vi "peis.vi"(0 "IP adress":string="192.109.209.229", 1 "stop":bool, 2 "Channel":u8(ring) items=["1", "2", "3", "4", "5", "6", "7", "8", "9", "10", "11", "12", "13", "14", "15", "16"], 3 "PEIS Parameters":T2={"Step_number"=0, "Initial_Voltage_step"=0.0, "vs_initial"=TRUE, "Final_Voltage_step"=1.0, "vs_final"=FALSE, "Duration_step"=1.0, "Record_every_dI"=0.1, "Record_every_dT"=0.1, "Initial_frequency"=100000.0, "sweep"=FALSE, "Final_frequency"=1.0, "Frequency_number"=51, "Amplitude_Voltage"=0.01, "Wait_for_steady"=2.0, "Average_N_times"=1, "Correction"=TRUE, "I_Range"=12, "Bandwidth"=5, "em"=1, "ce"=0} {"ce" items=["Standard", "CE to ground"]; "Initial_Voltage_step" min=-10 max=10 format="%.5f"; "Step_number" min=0 step=1; "I_Range" items=["1pA", "1nA", "10nA", "100nA", "1µA", "10µA", "100µA", "1mA", "10mA", "100mA", "1A", "Booster", "Auto"]; "Wait_for_steady" min=0 format="%.2f"; "Record_every_dT" min=0 format="%.2e"; "Record_every_dI" min=0 format="%.2e"; "Duration_step" min=0 format="%.5f"; "Final_Voltage_step" min=-10 max=10 format="%.5f"; "Bandwidth" items=["1"=1, "2"=2, "3"=3, "4"=4, "5"=5, "6"=6, "7"=7, "8"=8, "9"=9]; "Average_N_times" min=1 max=1000 step=1; "Amplitude_Voltage" min=0.0005 max=0.5 format="%.2e"; "Final_frequency" min=1e-05 max=1000000 format="%.2e"; "Frequency_number" min=1 max=10000; "Initial_frequency" min=1e-05 max=1000000 format="%.2e"}, 4 "Exit":bool, 5 "Start":bool, 8 "Draw":T1(ring)) -> (6 "XY Graph":cluster{"Data p1":sgl[], "Data p1":dbl[]}[](graph), 7 "Number of points":i32=52)   [LabVIEW 2016]
doc: "The Staircase Potentio Electrochemical Impedance Spectroscopy (SPEIS) technique is designed to perform successive impedance measurements (on a whole frequency range) during a potential sweep. \nThis technique consists in a staircase potential sweep (potential limits and number of steps defined by the user). An impedance measurement (with an adjustable number of frequencies) is performed on each potential step.\n\nIn general, in this VI, the first thing to do is to start by establishing the connection with the instrument defined by its IP adress, then load the firmware in the channel selected, get the information on the plugged channels, load protocol on a channel, start/stop the protocol, retreive data and draw the graph.\nThis technique is applied just for channels with impedance capabilities (Zboard)."
uses:
  LLB/dll_Functions.llb/PEISParameters.ctl
panel:
  in  "Display Parameters?":bool caption="Display Parameters"
  out "DllPath":path caption="DLL Path"
  out "LibVersion":string caption="DLL Version"
  out "Data p0":sgl[][](array[numeric])=[[0.100008, 0.099745475, 1.9343544e-05], [0.200016, 0.09966919, 1.936642e-05], [0.300024, 0.10005063, 1.9374045e-05], [0.400032, 0.10005063, 1.9358795e-05], [0.50004, 0.09997434, 1.9358795e-05], [0.600048, 0.09982177, 1.938167e-05], [0.700056, 0.099516615, 1.9358795e-05], [0.800064, 0.099898055, 1.9374045e-05], [0.90007204, 0.099516615, 1.936642e-05]]
  out "Data p1":sgl[][](array[numeric])=[[99999.99, 0.009897927, 1.5485124e-05, -0.23932889, 0.09957624, 2.0601647e-05, 0.0, 0.017584162, 1.5528842e-05, -0.13801742, -0.10928005, -2.0601661e-05, 0.0, 1.89, 7.0], [79789.055, 0.009909321, 1.4999416e-05, -0.28277892, 0.09956935, 2.0610883e-05, 0.0, 0.017358849, 1.5026583e-05, -0.16497254, -0.10927754, -2.0610896e-05, 0.0, 2.319, 7.0], [63671.867, 0.00993305, 1.4371862e-05, -0.3338619, 0.099571265, 2.0617736e-05, 0.0, 0.01701651, 1.4388475e-05, -0.19887781, -0.10927467, -2.0617748e-05, 0.0, 2.748, 7.0], [50804.684, 0.009895762, 1.349999e-05, -0.38682938, 0.099595726, 2.0621628e-05, 0.0, 0.016509676, 1.3509973e-05, -0.23511207, -0.10929042, -2.0621641e-05, 0.0, 3.177, 7.0], [40539.06, 0.009924297, 1.2531375e-05, -0.43154812, 0.09956674, 2.0623062e-05, 0.0, 0.01605967, 1.2537333e-05, -0.27001935, -0.1092824, -2.0623074e-05, 0.0, 3.606, 7.0], [32343.752, 0.009929493, 1.1422184e-05, -0.4605673, 0.099575475, 2.0627644e-05, 0.0, 0.015497766, 1.1425662e-05, -0.29694676, -0.10927959, -2.0627656e-05, 0.0, 4.035, 7.0], [25812.496, 0.009931898, 1.0332502e-05, -0.47349262, 0.09957423, 2.0616248e-05, 0.0, 0.014982226, 1.0334525e-05, -0.31350675, -0.10928383, -2.0616259e-05, 0.0, 4.4639997, 7.0], [20593.748, 0.009683827, 9.104932e-06, -0.46709442, 0.09957324, 2.0613099e-05, 0.0, 0.014134236, 9.106069e-06, -0.3174526, -0.10928545, -2.0613114e-05, 0.0, 4.75, 7.0], [16429.69, 0.00984061, 8.381006e-06, -0.4425385, 0.0995779, 2.0614962e-05, 0.0, 0.013980997, 8.381673e-06, -0.30736777, -0.10928426, -2.0614974e-05, 0.0, 5.036, 7.0], [13109.373, 0.009880392, 7.759602e-06, -0.4042132, 0.09956233, 2.0629059e-05, 0.0, 0.013766184, 7.759997e-06, -0.28469434, -0.10927877, -2.0629072e-05, 0.0, 5.322, 7.0], [10460.936, 0.009915135, 7.290463e-06, -0.35881066, 0.099576354, 2.062228e-05, 0.0, 0.013552605, 7.2907023e-06, -0.25464892, -0.10927802, -2.0622294e-05, 0.0, 5.608, 7.0], [8351.5625, 0.009958473, 6.968417e-06, -0.30687237, 0.09957134, 2.0619169e-05, 0.0, 0.013452288, 6.968562e-06, -0.21966934, -0.10928822, -2.0619183e-05, 0.0, 5.894, 7.0], [6660.1553, 0.009773157, 6.585265e-06, -0.26302314, 0.09957721, 2.0628519e-05, 0.0, 0.013077308, 6.5853465e-06, -0.18975565, -0.109301746, -2.0628531e-05, 0.0, 6.0620003, 7.0], [5313.953, 0.009875495, 6.4977903e-06, -0.21722555, 0.09959636, 2.061105e-05, 0.0, 0.013129692, 6.497844e-06, -0.15612268, -0.10930546, -2.0611064e-05, 0.0, 6.269, 7.0], [4241.786, 0.009916322, 6.4091464e-06, -0.17841792, 0.09959986, 2.0643229e-05, 0.0, 0.013149473, 6.4091746e-06, -0.12683374, -0.109303646, -2.0643243e-05, 0.0, 6.4830003, 7.0], [3385.4163, 0.009962957, 6.371731e-06, -0.15283132, 0.09959816, 2.0641255e-05, 0.0, 0.013166811, 6.371748e-06, -0.11219756, -0.10930573, -2.0641268e-05, 0.0, 6.697, 7.0], [2699.3184, 0.009985389, 6.3324687e-06, -0.12883663, 0.099599674, 2.0642745e-05, 0.0, 0.013169419, 6.3324833e-06, -0.09362733, -0.10931173, -2.0642758e-05, 0.0, 6.9110003, 7.0], [2153.4448, 0.009996085, 6.3133293e-06, -0.11305499, 0.09959159, 2.0643656e-05, 0.0, 0.013185124, 6.313335e-06, -0.08275235, -0.109307505, -2.064367e-05, 0.0, 7.125, 7.0], [1717.748, 0.010014333, 6.2567524e-06, -0.10080016, 0.09959457, 2.0655203e-05, 0.0, 0.013182044, 6.256763e-06, -0.07431483, -0.10931141, -2.0655216e-05, 0.0, 7.34, 7.0], [1372.1951, 0.010016238, 6.2877625e-06, -0.09321749, 0.09959682, 2.064688e-05, 0.0, 0.013175669, 6.2877634e-06, -0.06877315, -0.10931128, -2.0646892e-05, 0.0, 7.5550003, 7.0], [1096.7545, 0.010012516, 6.286433e-06, -0.08541584, 0.09960139, 2.0640491e-05, 0.0, 0.013178928, 6.2864306e-06, -0.062073976, -0.10930484, -2.0640506e-05, 0.0, 7.77, 7.0], [871.93097, 0.010010969, 6.268487e-06, -0.08781743, 0.09959833, 2.0634905e-05, 0.0, 0.013172707, 6.2684835e-06, -0.06440747, -0.109307244, -2.0634918e-05, 0.0, 7.987, 7.0], [696.1138, 0.01003125, 6.2508416e-06, -0.093888, 0.09959319, 2.0650714e-05, 0.0, 0.013164024, 6.2508466e-06, -0.069969416, -0.10931639, -2.0650728e-05, 0.0, 8.203, 7.0], [555.8894, 0.010025321, 6.2520185e-06, -0.10746312, 0.099596396, 2.063822e-05, 0.0, 0.01315077, 6.2520166e-06, -0.08037281, -0.109306626, -2.0638234e-05, 0.0, 8.42, 7.0], [443.43906, 0.010033136, 6.209101e-06, -0.12175393, 0.0995993, 2.0631758e-05, 0.0, 0.01312816, 6.2091035e-06, -0.091670275, -0.109299496, -2.063177e-05, 0.0, 8.639, 7.0], [353.75473, 0.01003465, 6.1840165e-06, -0.14335668, 0.09959073, 2.0645593e-05, 0.0, 0.013097799, 6.1840187e-06, -0.10758209, -0.10931424, -2.0645608e-05, 0.0, 8.859, 7.0], [281.8943, 0.010030967, 6.109471e-06, -0.17281115, 0.09959446, 2.0650212e-05, 0.0, 0.013065848, 6.109473e-06, -0.129511, -0.10930905, -2.0650225e-05, 0.0, 9.0789995, 7.0], [225.3606, 0.010023677, 6.0119432e-06, -0.20512176, 0.09959748, 2.064375e-05, 0.0, 0.013001974, 6.0119396e-06, -0.15545309, -0.1093129, -2.0643763e-05, 0.0, 9.301, 7.0], [180.28844, 0.010028235, 5.913567e-06, -0.25207758, 0.0995884, 2.0643136e-05, 0.0, 0.012923154, 5.913563e-06, -0.19031943, -0.1093126, -2.0643149e-05, 0.0, 9.526, 7.0], [143.75787, 0.010025335, 5.723294e-06, -0.2980666, 0.09959362, 2.0638052e-05, 0.0, 0.012791262, 5.7232987e-06, -0.22673774, -0.109312676, -2.0638066e-05, 0.0, 9.755, 7.0], [114.59661, 0.0100282775, 5.478785e-06, -0.36026663, 0.09959826, 2.0642558e-05, 0.0, 0.012615283, 5.4787893e-06, -0.27884817, -0.109307505, -2.0642572e-05, 0.0, 9.987, 7.0], [91.552734, 0.010020258, 5.1631105e-06, -0.41180015, 0.09958356, 2.0632298e-05, 0.0, 0.012400166, 5.1631077e-06, -0.32256132, -0.10930771, -2.0632311e-05, 0.0, 10.219, 7.0], [72.87778, 0.010045694, 4.7920767e-06, -0.47027957, 0.0995903, 1.9318108e-05, 0.0, 0.012195916, 4.7920753e-06, -0.37585485, -0.10930665, -1.931812e-05, 0.0, 10.735, 6.0], [58.30223, 0.010017018, 4.3459513e-06, -0.5196618, 0.09958969, 1.931711e-05, 0.0, 0.011869716, 4.345951e-06, -0.41790736, -0.109305374, -1.9317124e-05, 0.0, 10.989, 6.0], [46.50297, 0.010043655, 3.8964367e-06, -0.5461425, 0.09958527, 1.9321726e-05, 0.0, 0.011661541, 3.8964395e-06, -0.45622373, -0.10929812, -1.9321737e-05, 0.0, 11.24, 6.0], [36.95101, 0.0100237075, 3.4589034e-06, -0.55786407, 0.09959118, 1.9322812e-05, 0.0, 0.011445447, 3.4589052e-06, -0.47548974, -0.1093029, -1.9322824e-05, 0.0, 11.498, 6.0], [29.592804, 0.010024518, 3.0782626e-06, -0.5442606, 0.099590674, 1.9320825e-05, 0.0, 0.011281099, 3.0782635e-06, -0.4723431, -0.10930497, -1.9320838e-05, 0.0, 11.782001, 6.0], [23.588463, 0.010025413, 2.7635026e-06, -0.50970626, 0.09959939, 1.931987e-05, 0.0, 0.011168829, 2.7635024e-06, -0.45203626, -0.10930516, -1.9319881e-05, 0.0, 12.092, 6.0], [18.780045, 0.010028319, 2.5114025e-06, -0.46162716, 0.0995976, 1.9318664e-05, 0.0, 0.01109292, 2.5114036e-06, -0.4128492, -0.109315775, -1.9318675e-05, 0.0, 12.425, 6.0], [15.024037, 0.010029642, 2.331001e-06, -0.4064955, 0.099582985, 1.9321948e-05, 0.0, 0.01104459, 2.3310024e-06, -0.36793888, -0.10930361, -1.9321958e-05, 0.0, 12.772, 6.0], [11.982363, 0.010013976, 2.1986236e-06, -0.3445742, 0.0995901, 1.9318428e-05, 0.0, 0.01101896, 2.198625e-06, -0.31417423, -0.10929007, -1.931844e-05, 0.0, 13.119, 6.0], [9.574144, 0.010021789, 2.1110484e-06, -0.29042864, 0.09959056, 1.931938e-05, 0.0, 0.011009957, 2.1110482e-06, -0.26570365, -0.10930588, -1.9319392e-05, 0.0, 13.55, 6.0], [7.6293964, 0.010015764, 2.047544e-06, -0.2358973, 0.09959619, 1.9324216e-05, 0.0, 0.010986972, 2.0475438e-06, -0.21676749, -0.10930043, -1.9324229e-05, 0.0, 14.088, 6.0], [6.084501, 0.010008753, 2.0095065e-06, -0.19609833, 0.09960107, 1.9321422e-05, 0.0, 0.010978085, 2.0095063e-06, -0.17923641, -0.10930903, -1.9321435e-05, 0.0, 14.758, 6.0], [4.858519, 0.0100127505, 1.9834858e-06, -0.15383446, 0.099605374, 1.9325236e-05, 0.0, 0.01099137, 1.983485e-06, -0.14275539, -0.10930968, -1.9325249e-05, 0.0, 15.594, 6.0], [3.8752477, 0.010018873, 1.964741e-06, -0.12660927, 0.09960577, 1.9319072e-05, 0.0, 0.01098087, 1.9647398e-06, -0.11773729, -0.10930894, -1.9319084e-05, 0.0, 16.639, 6.0], [3.1001983, 0.01002199, 1.954336e-06, -0.101673305, 0.09960291, 1.9318823e-05, 0.0, 0.010977447, 1.9543347e-06, -0.09406805, -0.10931086, -1.9318833e-05, 0.0, 17.943, 6.0], [2.4660668, 0.010017678, 1.9471984e-06, -0.08063111, 0.09960053, 1.9318097e-05, 0.0, 0.010982101, 1.9471975e-06, -0.07494378, -0.10931104, -1.9318108e-05, 0.0, 19.579, 6.0], [1.9649143, 0.01001538, 1.9460967e-06, -0.064157724, 0.09960199, 1.9316354e-05, 0.0, 0.010980325, 1.946096e-06, -0.06017399, -0.1093061, -1.9316365e-05, 0.0, 21.627, 6.0], [1.5725644, 0.010012327, 1.941652e-06, -0.051375534, 0.09960348, 1.9317453e-05, 0.0, 0.010977772, 1.9416514e-06, -0.04843211, -0.10930792, -1.9317464e-05, 0.0, 24.183, 6.0], [1.2520034, 0.010019626, 1.939335e-06, -0.041469768, 0.09961237, 1.9318904e-05, 0.0, 0.010981496, 1.9393347e-06, -0.038478374, -0.109313786, -1.9318915e-05, 0.0, 27.391, 6.0], [1.0016024, 0.010014649, 1.938777e-06, -0.033258826, 0.09960662, 1.931856e-05, 0.0, 0.010977961, 1.9387764e-06, -0.031450033, -0.109310396, -1.9318572e-05, 0.0, 31.398, 6.0]]
  out "Exit 2":bool=TRUE
  # "Instructions:\nBefore running the VI you must type a valid IP adress that corresponds to the instrument.Then press the Run button to execute this VI.\nWhile this VI is running, choose the available channel, enter the SPEIS parameters or keep the default\n values, then press the start button to begin the experience. \nChoose the waveform to draw : Nyquist, modZ, theta...\nPress the stop button to end experience and the exit button to stop the VI execution."
  # "Set E (V)  vs. previous"
  # "Before EIS  stay for ts (s)"
  # "and record every dI (A)"
  # "or every dt (s)"
  # "Start EIS from  Fi (Hz)"
  # "sweep linear/logarithmic"
  # "to Ff (Hz)"
  # "for Nf frequencies"
  # "with the amplitude (V)"
  # "wait for Pw"
  # "average Na times"
  # "drift correction"
  # "with I Range"
  # "and bandwidth"
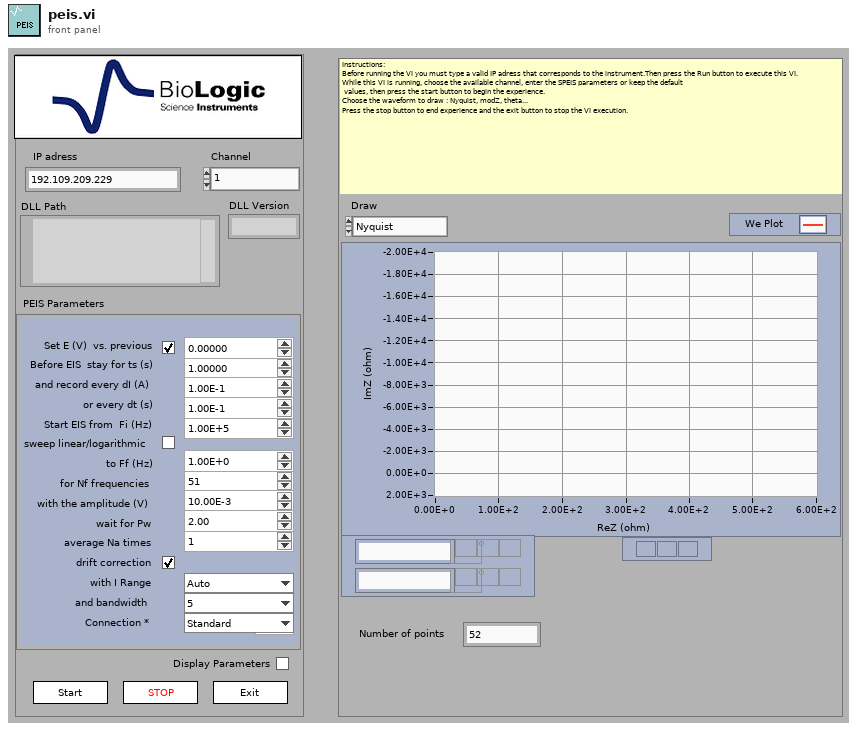
[diagram p1: front panel]
types:
  T1 = enum16{"Nyquist", "modZ", "theta", "modE", "modI", "Edc", "Idc", "E range", "I range", "f(t)"}
  T2 = typedef "PEISParameters.ctl" = cluster{"Step_number":i32, "Initial_Voltage_step":sgl, "vs_initial":bool, "Final_Voltage_step":sgl, "vs_final":bool, "Duration_step":sgl, "Record_every_dI":sgl, "Record_every_dT":sgl, "Initial_frequency":sgl, "sweep":bool, "Final_frequency":sgl, "Frequency_number":i32, "Amplitude_Voltage":sgl, "Wait_for_steady":sgl, "Average_N_times":i32, "Correction":bool, "I_Range":u16, "Bandwidth":u16, "em":u16, "ce":u16}
  T3 = cluster{"LibVersion":string, "StringLength":u32, "DllPath":path}
  T4 = cluster{"Channel":i32, "BoardVersion":i32, "BoardSerialCode":i32, "FirmwareCode":i32, "FirmwareVersion":i32, "XilinxVersion":i32, "AmpCode":i32, "NbAmp":i32, "LcBoard":i32, "Zboard":i32, "MuxBoard":i32, "GPRAboard":i32, "MemSize":i32, "MemFilled":i32, "state":i32, "MaxIRange":i32, "MinIRange":i32, "MaxBandwidth":i32, "NbOfTechniques":i32}
  T5 = typedef "TechniqueParameters.ctl" = cluster{"String Label":string, "Type":i32, "Valeur":i32, "Index":i32}
  T6 = cluster{"string before end tag":string, i32, i32, i32}[]
  T7 = cluster{"IRQskipped":i32, "NbRaws":i32, "NbCols":i32, "Technique Index":i32, "TechniqueID":i32, "PrcessIndex":i32, "loop":i32, "StartTime":dbl, "MuxPad":i32}
  T8 = cluster{"State":i32, "MemFilled":i32, "TimeBase":sgl, " Ewe":sgl, " EweRangeMin":sgl, " EweRangeMax":sgl, "Ece":sgl, "EceRangeMin":sgl, "EceRangeMax":sgl, "Eoverflow":i32, "I":sgl, "IRange":i32, "Ioverflow":i32, "ElapsedTime":sgl, "Freq":sgl, "Rcomp":sgl, "Saturation":sgl, "OptErr":i32, "OptPos":i32}
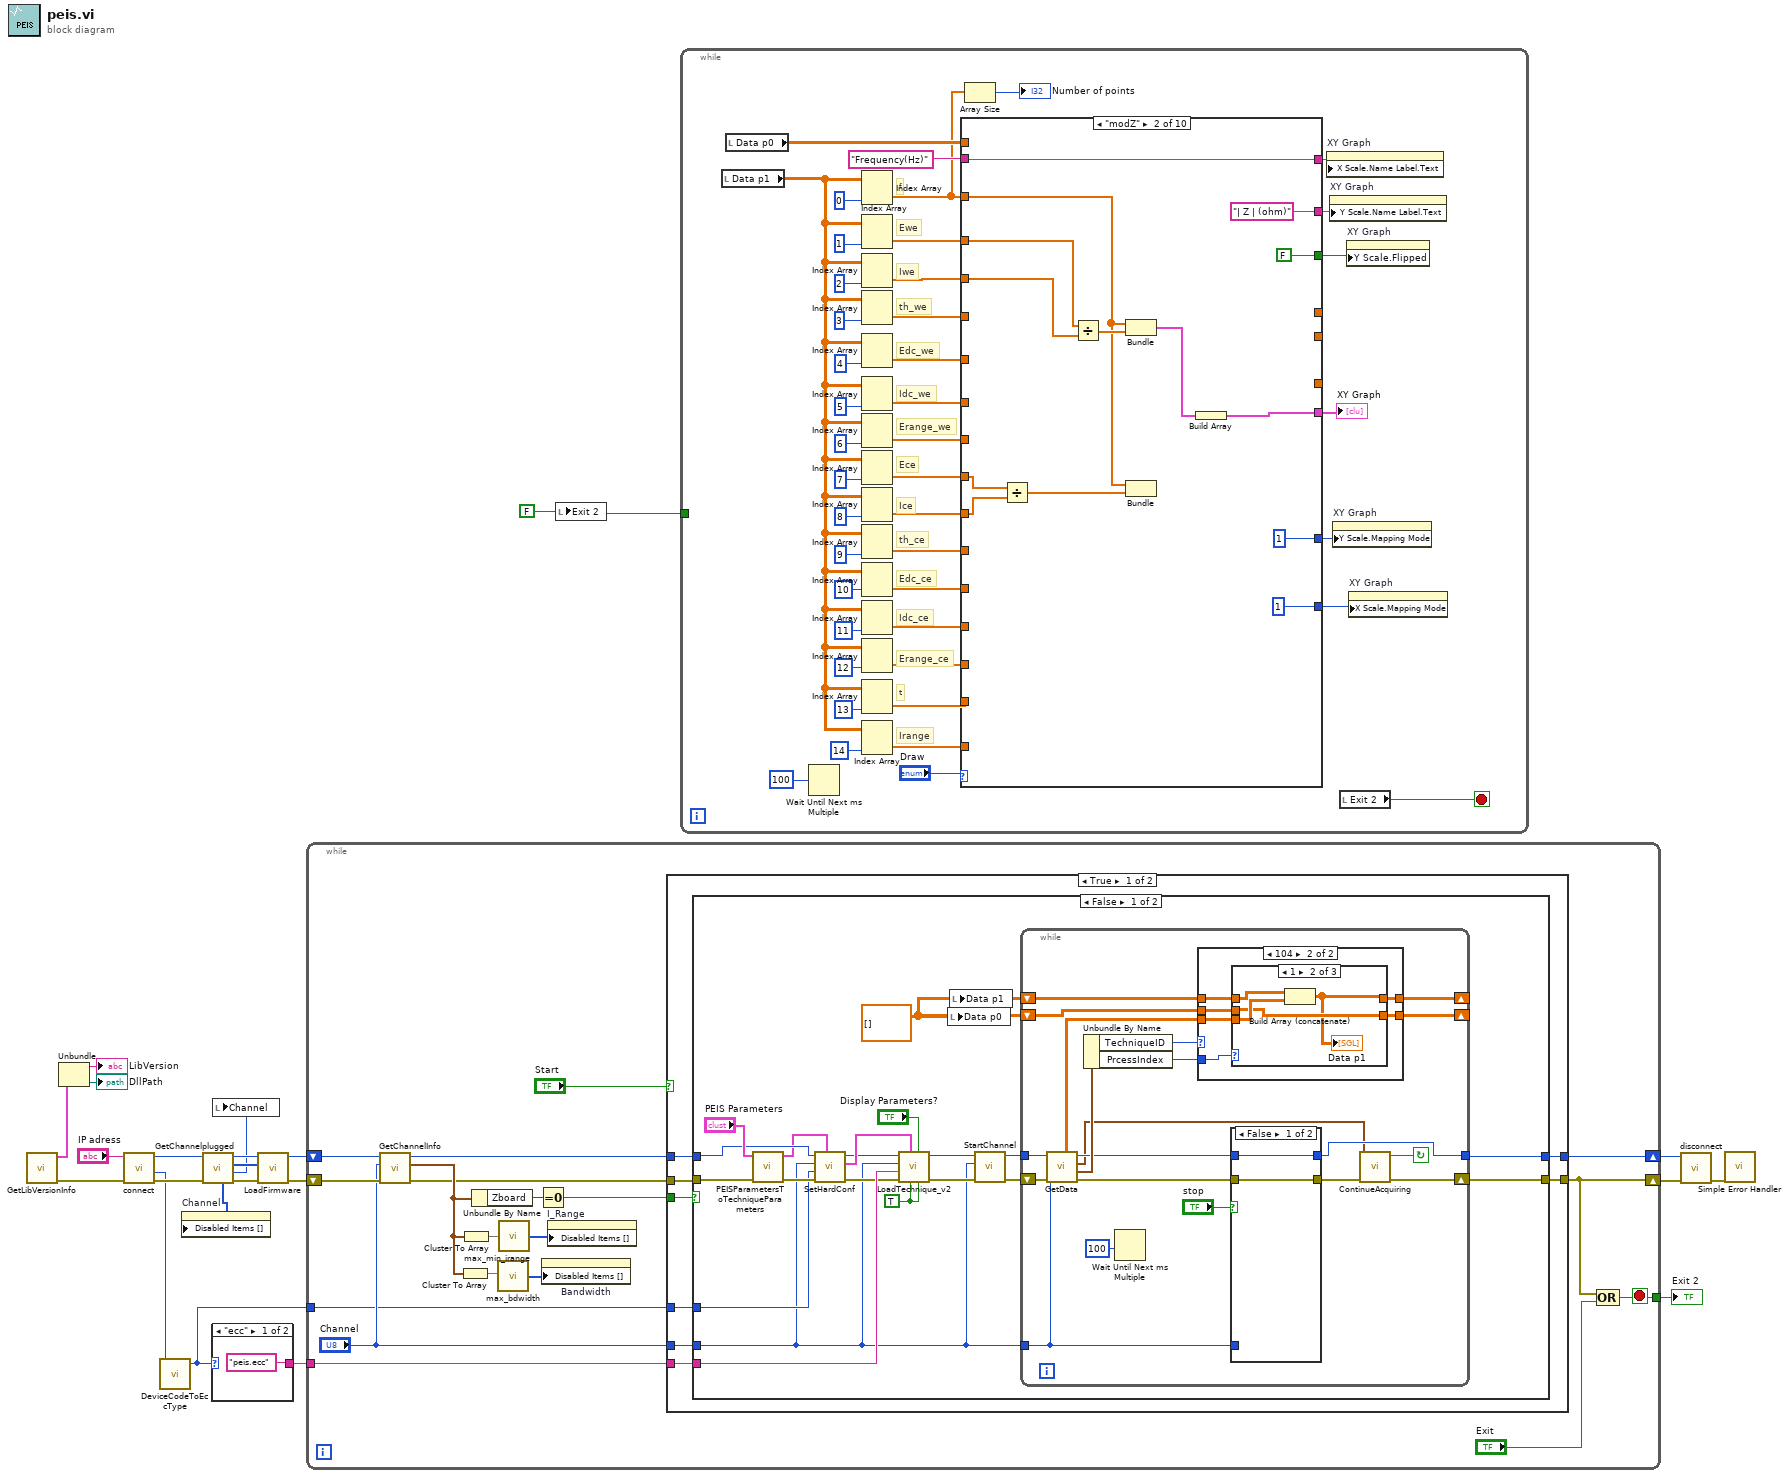
[diagram p0: block diagram]
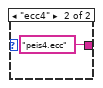
[diagram p2: hidden frame]
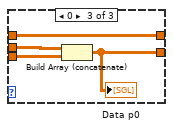
[diagram p5: hidden frame]
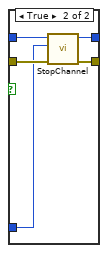
[diagram p6: hidden frame]
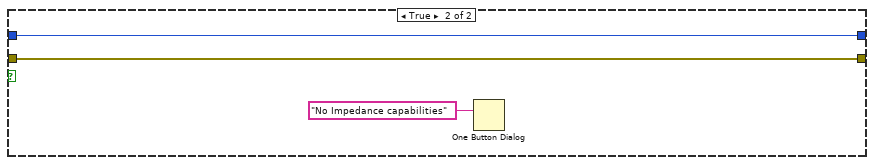
[diagram p7: hidden frame]
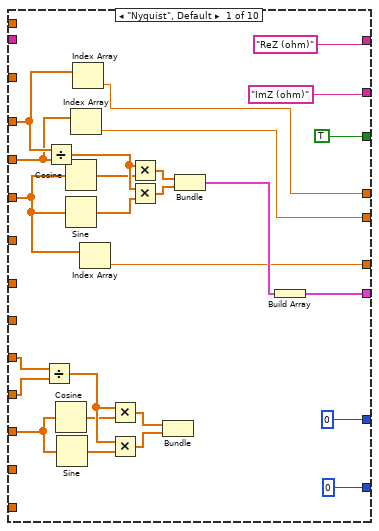
[diagram p9: hidden frame]
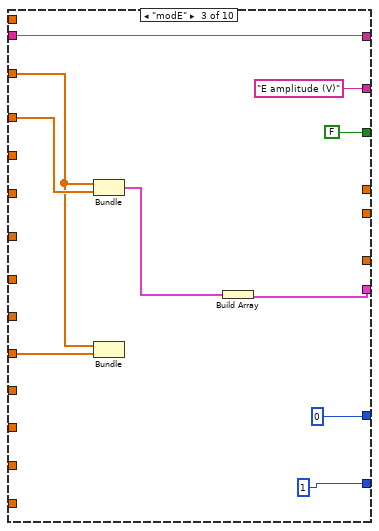
[diagram p10: hidden frame]
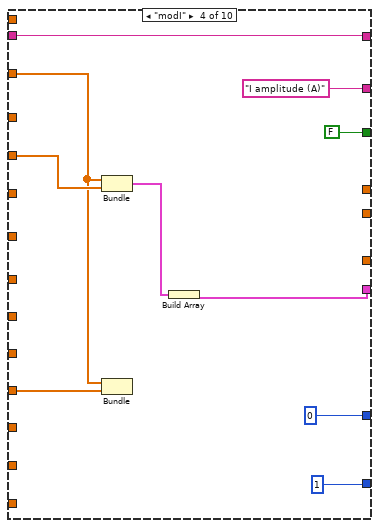
[diagram p11: hidden frame]
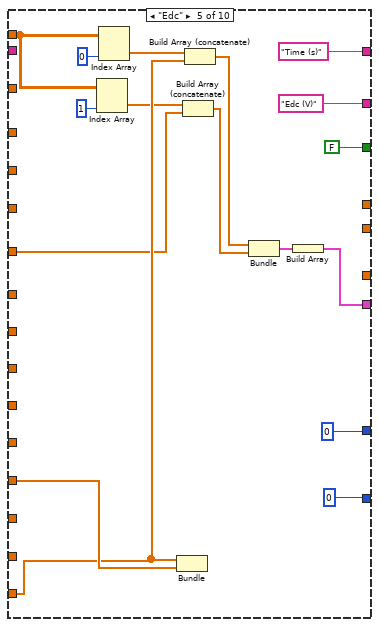
[diagram p12: hidden frame]
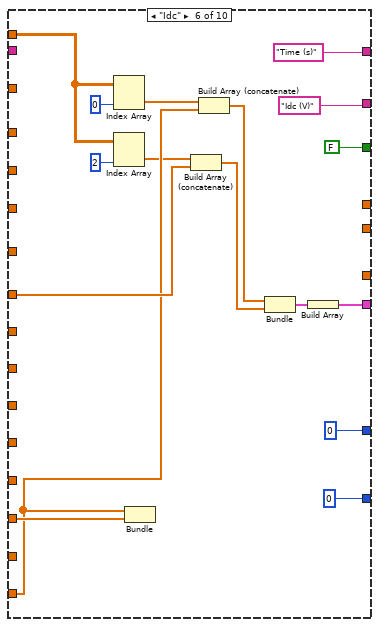
[diagram p13: hidden frame]
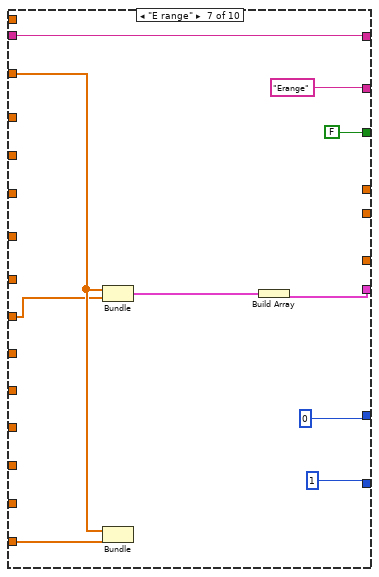
[diagram p14: hidden frame]
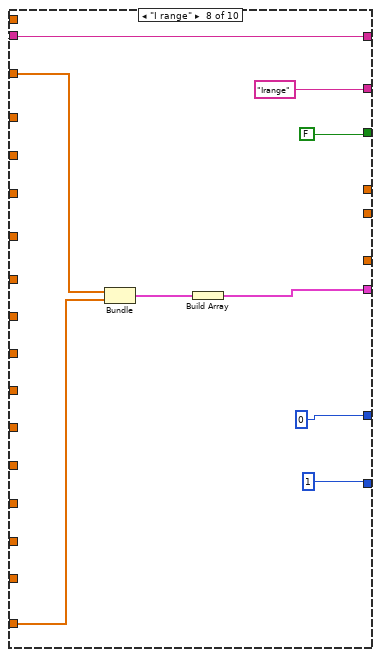
[diagram p15: hidden frame]
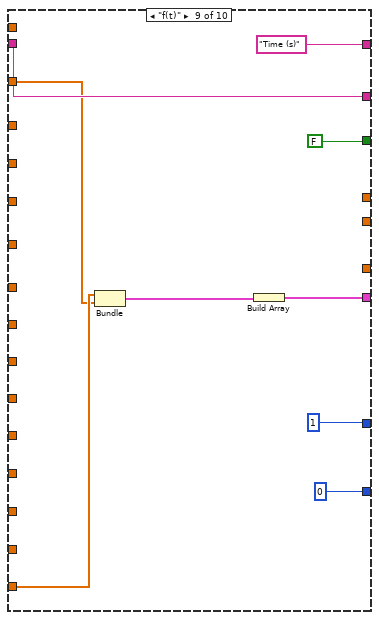
[diagram p16: hidden frame]
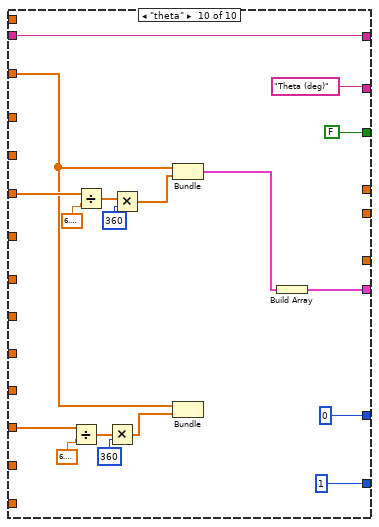
[diagram p17: hidden frame]
diagram:
  w21 = FALSE
  n1 = call "GetLibVersionInfo.vi"() -> ("error out"=w1:errorcluster, "LibInfo"=w4:T3)  [unwired: 10 in]
  n2 = Unbundle(w4) -> ("LibVersion"=→"LibVersion":string, "DllPath"=→"DllPath":path)  [unwired: 1 out]
  n3 = call "connect.vi"("error in (no error)"=w1, "IP"="IP adress") -> ("error out"=w18:errorcluster, "Device Code"=w10:i32, "ID Out"=w20:i32)  [unwired: 6 in, 1 out]
  n4 = call "DeviceCodeToEccType.vi"("Device Code"=w10) -> ("EccType"=w5:enum16{"ecc", "ecc4"})  [unwired: 4 in]
  n5 = call "GetChannelplugged.vi"("error in (no error)"=w18, "ID In"=w20) -> ("error out"=w17:errorcluster, "FirstPluggedChannel"=w6:u8, "PluggedChannels"=w15:u8[], "ID Out"=w14:i32, "DisabledChannels"=w16:i32[])  [unwired: 5 in]
  n6 = property on="Channel" class="Ring (strict)"("Disabled Items []"=w16) -> ()  [unwired: 2 in, 2 out]
  n7 = case shown="\"ecc\"" w5 {
    tunnel: ["peis.ecc" ("FName") "peis4.ecc" ("FName")] -> w9
    frame "ecc" {
    }
    frame "ecc4" {
    }
  }
  n8 = local write "Channel"(w6) -> ()
  n9 = call "LoadFirmware.vi"("error in (no error)"=w17, "Channels"=w15, "ID In"=w14) -> ("error out"=w13:errorcluster, "ID Out"=w12:i32)  [unwired: 6 in, 1 out]
  n10 = while {
    shift-right: [w28] -> w11
    shift-left: w13 -> [w35]
    tunnel: w9 -> [w29]
    shift-right: [w36] -> w19
    shift-left: w12 -> [w34]
    tunnel: [w26] -> w7
    tunnel: w5 -> [w25]
    stop <- w26 stop-if-true
    n11 = call "GetChannelInfo.vi"("error in (no error)"=w35, "Channel"="Channel", "ID"=w34) -> ("error out"=w30:errorcluster, "Channel information"=w32:T4, "ID Out"=w31:i32)  [unwired: 6 in]
    n12 = Cluster To Array(cluster=w32) -> (array=w39:i32[])
    n13 = Cluster To Array(cluster=w32) -> (array=w42:i32[])
    n14 = Unbundle By Name(w32) -> ("Zboard"=w41:i32)
    n15 = call "max_bdwidth.vi"("resources"=w39) -> ("disabled ranges"=w38:i32[])
    n16 = call "max_min_irange.vi"("resources"=w42) -> ("disabled ranges"=w37:i32[])
    n17 = Equal To 0?(x=w41) -> (x = 0?=w40:bool)
    n18 = property on="Bandwidth" class="Ring (strict)"("Disabled Items []"=w38) -> ()  [unwired: 2 in, 2 out]
    n19 = property on="I_Range" class="Ring (strict)"("Disabled Items []"=w37) -> ()  [unwired: 2 in, 2 out]
    n20 = case shown="True" "Start" {
      tunnel: "Channel" -> [w50 _]
      tunnel: [w51 w121] -> w28
      tunnel: w30 -> [w49 w121]
      tunnel: w40 -> [w48 _]
      tunnel: w31 -> [w47 w120]
      tunnel: [w46 w120] -> w36
      tunnel: w29 -> [w45 _]
      tunnel: w25 -> [w44 _]
      frame True {
        n21 = case shown="False" w48 {
          tunnel: [w71 w118] -> w51
          tunnel: w50 -> [w53 _]
          tunnel: w49 -> [w67 w118]
          tunnel: w47 -> [w56 w117]
          tunnel: [w62 w117] -> w46
          tunnel: w45 -> [w64 _]
          tunnel: w44 -> [w54 _]
          frame False {
            w61 = TRUE ("First Protocol")
            w70 = sgl[][] [] ("Data")
            n22 = call "PEISParametersToTechniqueParameters.vi"("error in (no error)"=w67, "PEIS Parameters"="PEIS Parameters") -> ("error out"=w60:errorcluster, "TechniqueParameters"=w55:T5[])  [unwired: 8 in]
            n23 = call "SetHardConf.vi"("Params Values"=w55, "error in (no error)"=w60, "EccType"=w54, "Channel"=w53, "ID In"=w56) -> ("error out"=w59:errorcluster, "Params Values Trimed"=w58:T6, "ID Out"=w57:i32)  [unwired: 4 in]
            n24 = call "LoadTechnique_v2.vi"("Last Protocol"=w61, "Display Parameters?"="Display Parameters?", "First Protocol"=w61, "TechniqueParameters"=w58, "error in (no error)"=w59, "FName"=w64, "Selected Channel"=w53, "ID In"=w57) -> ("error out"=w66:errorcluster, "ID  Out"=w65:i32)  [unwired: 2 in]
            n25 = local write "Data p0"(w70) -> ()
            n26 = local write "Data p1"(w70) -> ()
            n27 = call "StartChannel.vi"("error in (no error)"=w66, "Channel"=w53, "ID In"=w65) -> ("error out"=w68:errorcluster, "ID Out"=w63:i32)  [unwired: 7 in]
            n28 = while {
              shift-right: [w77] -> w71
              shift-left: w68 -> [w91]
              shift-right: [w86] -> _
              shift-left: w70 -> [w87]
              shift-right: [w85] -> _
              shift-left: w70 -> [w84]
              tunnel: w53 -> [w78]
              tunnel: w63 -> [w81]
              tunnel: [w79] -> w62
              stop <- w88 continue-if-true
              n29 = call "GetData.vi"("error in (no error)"=w91, "Channel"=w78, "ID In"=w81) -> ("error out"=w89:errorcluster, "Data information"=w82:T7, "Current values"=w73:T8, "ID Out"=w80:i32, "Data"=w74:dbl[][])  [unwired: 4 in]
              n30 = Unbundle By Name(w82) -> ("TechniqueID"=w75:i32, "PrcessIndex"=w72:i32)
              n31 = Wait Until Next ms Multiple(millisecond multiple=u32 100) -> ()  [unwired: 1 out]
              n32 = case shown="104" w75 {
                tunnel: w74 -> [_ w99]
                tunnel: w87 -> [w93 w98]
                tunnel: [w93 w97] -> w86
                tunnel: [w92 w96] -> w85
                tunnel: w84 -> [w92 w95]
                tunnel: w72 -> [_ w94]
                frame Default {
                }
                frame 104 {
                  n33 = case shown="1" w94 {
                    tunnel: w99 -> [_ w105 w109]
                    tunnel: w98 -> [w101 w104 w107]
                    tunnel: [w101 w102 w107] -> w97
                    tunnel: [w100 w103 w106] -> w96
                    tunnel: w95 -> [w100 w103 w108]
                    frame Default {
                    }
                    frame 1 {
                      n34 = Build Array (concatenate)(w104, w105) -> (w102:dbl[][])
                      "Data p1" <- w102
                    }
                    frame 0 {
                      n35 = Build Array (concatenate)(w108, w109) -> (w106:dbl[][])
                      "Data p0" <- w106
                    }
                  }
                }
              }
              n36 = case shown="False" "stop" {
                tunnel: [w111 w116] -> w76
                tunnel: w89 -> [w111 w115]
                tunnel: w80 -> [w110 w114]
                tunnel: [w110 w113] -> w79
                tunnel: w78 -> [_ w112]
                frame False {
                }
                frame True {
                  n37 = call "StopChannel.vi"("error in (no error)"=w115, "Channel"=w112, "ID In"=w114) -> ("error out"=w116:errorcluster, "ID Out"=w113:i32)  [unwired: 7 in]
                }
              }
              n38 = call "ContinueAcquiring.vi"("error in"=w76, "Current values"=w73) -> ("error out"=w77:errorcluster, "ContinueAcquiring?"=w88:bool)  [unwired: 8 in]
            }
          }
          frame True {
            n39 = One Button Dialog(message="No Impedance capabilities" ("error source (\" \")")) -> ()  [unwired: 1 in, 1 out]
          }
        }
      }
      frame False {
      }
    }
    n40 = Compound Arithmetic op=OR(w28, "Exit") -> (w26:bool)
  }
  "Exit 2" <- w7
  n41 = local write "Exit 2"(w21) -> ()
  n42 = while {
    tunnel: w21 -> [_]
    stop <- w153 stop-if-true
    # "Erange_ce"
    # "Idc_ce"
    # "Edc_ce"
    # "th_ce"
    # "Ice"
    # "Ece"
    # "t"
    # "Irange"
    # "Erange_we"
    # "Idc_we"
    # "Edc_we"
    # "th_we"
    # "Iwe"
    # "Ewe"
    # "f"
    n43 = local read "Data p1"() -> (w138:sgl[][])
    n44 = local read "Data p0"() -> (w125:sgl[][])
    n45 = Wait Until Next ms Multiple(millisecond multiple=u32 100) -> ()  [unwired: 1 out]
    n46 = Index Array(array=w138, index (col)=0 ("Index")) -> (element=w124:sgl[])  [unwired: 1 in]
    n47 = Index Array(array=w138, index (col)=1 ("Index")) -> (element=w139:sgl[])  [unwired: 1 in]
    n48 = Index Array(array=w138, index (col)=2 ("Index")) -> (element=w143:sgl[])  [unwired: 1 in]
    n49 = Index Array(array=w138, index (col)=3 ("Index")) -> (element=w158:sgl[])  [unwired: 1 in]
    n50 = Index Array(array=w138, index (col)=4 ("disabled index (col)")) -> (element=w152:sgl[])  [unwired: 1 in]
    n51 = Index Array(array=w138, index (col)=5 ("disabled index (col)")) -> (element=w149:sgl[])  [unwired: 1 in]
    n52 = Index Array(array=w138, index (col)=6 ("index (row)")) -> (element=w140:sgl[])  [unwired: 1 in]
    n53 = Index Array(array=w138, index (col)=7) -> (element=w131:sgl[])  [unwired: 1 in]
    n54 = Index Array(array=w138, index (col)=8) -> (element=w130:sgl[])  [unwired: 1 in]
    n55 = Index Array(array=w138, index (col)=9) -> (element=w129:sgl[])  [unwired: 1 in]
    n56 = Index Array(array=w138, index (col)=10) -> (element=w128:sgl[])  [unwired: 1 in]
    n57 = Index Array(array=w138, index (col)=11) -> (element=w127:sgl[])  [unwired: 1 in]
    n58 = Index Array(array=w138, index (col)=12) -> (element=w126:sgl[])  [unwired: 1 in]
    n59 = Index Array(array=w138, index (col)=13 ("disabled index (col)")) -> (element=w141:sgl[])  [unwired: 1 in]
    n60 = Index Array(array=w138, index (col)=14 ("disabled index (col)")) -> (element=w142:sgl[])  [unwired: 1 in]
    n61 = case shown="\"modZ\"" "Draw" {
      tunnel: w124 -> [_ w193 w207 w218 _ _ w263 w271 w280 w289]
      tunnel: w139 -> [w169 w204 w214 _ _ _ _ _ _ _]
      tunnel: w143 -> [w168 w197 _ w224 _ _ _ _ _ _]
      tunnel: ["ImZ (ohm)" ("Y Scale.Name Label.Text") "| Z | (ohm)" ("Y Scale.Name Label.Text") "E amplitude (V)" ("Y Scale.Name Label.Text") "I amplitude (A)" ("Y Scale.Name Label.Text") "Edc (V)" ("Y Scale.Name Label.Text") "Idc (V)" ("Y Scale.Name Label.Text") "Erange" ("Y Scale.Name Label.Text") "Irange" ("Y Scale.Name Label.Text") w285 "Theta (deg)" ("Y Scale.Name Label.Text")] -> w160
      tunnel: w158 -> [w170 _ _ _ _ _ _ _ _ w298]
      tunnel: ["ReZ (ohm)" ("Y Scale.Name Label.Text") w201 w212 w222 "Time (s)" ("Y Scale.Name Label.Text") "Time (s)" ("Y Scale.Name Label.Text") w268 w277 "Time (s)" ("Y Scale.Name Label.Text") w304] -> w157
      tunnel: "Frequency(Hz)" ("Y Scale.Name Label.Text") -> [_ w201 w212 w222 _ _ w268 w277 w285 w304]
      tunnel: [TRUE ("Y Scale.Flipped") FALSE ("Y Scale.Flipped") FALSE ("Y Scale.Flipped") FALSE ("Y Scale.Flipped") FALSE ("Y Scale.Flipped") FALSE ("Y Scale.Flipped") FALSE ("Y Scale.Flipped") FALSE FALSE FALSE ("Y Scale.Flipped")] -> w155
      tunnel: [u8 0 ("X Scale.Mapping Mode") u8 1 ("X Scale.Mapping Mode") u8 1 ("X Scale.Mapping Mode") u8 1 ("X Scale.Mapping Mode") 0 0 1 1 0 u8 1 ("X Scale.Mapping Mode")] -> w154
      tunnel: w152 -> [_ _ _ _ w225 _ _ _ _ _]
      tunnel: w149 -> [_ _ _ _ _ w246 _ _ _ _]
      tunnel: w140 -> [_ _ _ _ _ _ w259 _ _ _]
      tunnel: w142 -> [_ _ _ _ _ _ _ w272 _ _]
      tunnel: w141 -> [_ _ _ _ w227 w245 _ _ w281 _]
      tunnel: [0 1 u8 0 ("X Scale.Mapping Mode") u8 0 ("X Scale.Mapping Mode") 0 0 0 0 1 0 ("X Scale.Mapping Mode")] -> w145
      tunnel: w131 -> [w182 w195 w208 _ _ _ _ _ _ _]
      tunnel: w130 -> [w181 w194 _ w217 _ _ _ _ _ _]
      tunnel: w129 -> [w180 _ _ _ _ _ _ _ _ w290]
      tunnel: w128 -> [_ _ _ _ w237 _ _ _ _ _]
      tunnel: w127 -> [_ _ _ _ _ w254 _ _ _ _]
      tunnel: w126 -> [_ _ _ _ _ _ w260 _ _ _]
      tunnel: [w175 w191 w205 w215 w236 w252 w261 w269 w278 w287] -> w122
      tunnel: w125 -> [_ _ _ _ w230 w248 _ _ _ _]
      tunnel: [w167 _ _ _ _ _ _ _ _ _] -> _
      tunnel: [w166 _ _ _ _ _ _ _ _ _] -> _
      tunnel: [w165 _ _ _ _ _ _ _ _ _] -> _
      frame "Nyquist", Default {
        n62 = Divide(x=w182, y=w181) -> (x/y=w177:sgl[])
        n63 = Divide(x=w169, y=w168) -> (x/y=w178:sgl[])
        n64 = Cosine(x=w180) -> (cos(x)=w176:sgl[])
        n65 = Sine(x=w180) -> (sin(x)=w183:sgl[])
        n66 = Cosine(x=w170) -> (cos(x)=w171:sgl[])
        n67 = Sine(x=w170) -> (sin(x)=w174:sgl[])
        n68 = Index Array(array=w168) -> (element=w167:sgl)  [unwired: 1 in]
        n69 = Index Array(array=w169) -> (element=w166:sgl)  [unwired: 1 in]
        n70 = Index Array(array=w170) -> (element=w165:sgl)  [unwired: 1 in]
        n71 = Multiply(x=w177, y=w176) -> (x*y=w185:sgl[])
        n72 = Multiply(x=w177, y=w183) -> (x*y=w184:sgl[])
        n73 = Multiply(x=w178, y=w171) -> (x*y=w173:sgl[])
        n74 = Multiply(x=w178, y=w174) -> (x*y=w172:sgl[])
        n75 = Bundle(w185, w184) -> ()  [unwired: 1 in, 1 out]
        n76 = Bundle(w173, w172) -> (w179:cluster{sgl[], sgl[]})  [unwired: 1 in]
        n77 = Build Array(w179) -> (w175:cluster{sgl[], sgl[]}[])
      }
      frame "modZ" {
        n78 = Divide(x=w195, y=w194) -> (x/y=w196:sgl[])
        n79 = Divide(x=w204, y=w197) -> (x/y=w203:sgl[])
        n80 = Bundle("Data p1"=w193, w203) -> (w192:cluster{"Data p1":sgl[], sgl[]})  [unwired: 1 in]
        n81 = Bundle("Data p1"=w193, w196) -> ()  [unwired: 1 in, 1 out]
        n82 = Build Array(w192) -> (w191:cluster{"Data p1":sgl[], sgl[]}[])
      }
      frame "modE" {
        n83 = Bundle("Data p1"=w207, "Data p1"=w214) -> (w206:cluster{"Data p1":sgl[], "Data p1":sgl[]})  [unwired: 1 in]
        n84 = Bundle("Data p1"=w207, "Data p1"=w208) -> ()  [unwired: 1 in, 1 out]
        n85 = Build Array(w206) -> (w205:cluster{"Data p1":sgl[], "Data p1":sgl[]}[])
      }
      frame "modI" {
        n86 = Bundle("Data p1"=w218, "Data p1"=w224) -> (w216:cluster{"Data p1":sgl[], "Data p1":sgl[]})  [unwired: 1 in]
        n87 = Bundle("Data p1"=w218, "Data p1"=w217) -> ()  [unwired: 1 in, 1 out]
        n88 = Build Array(w216) -> (w215:cluster{"Data p1":sgl[], "Data p1":sgl[]}[])
      }
      frame "Edc" {
        n89 = Index Array(array=w230, index (col)=1 ("Index")) -> (element=w226:sgl[])  [unwired: 1 in]
        n90 = Index Array(array=w230, index (col)=0 ("Index")) -> (element=w228:sgl[])  [unwired: 1 in]
        n91 = Bundle("Data p1"=w227, "Data p1"=w237) -> ()  [unwired: 1 in, 1 out]
        n92 = Build Array (concatenate)(w226, w225) -> (w232:sgl[])
        n93 = Build Array (concatenate)(w228, w227) -> (w233:sgl[])
        n94 = Bundle(w233, w232) -> (w229:cluster{sgl[], sgl[]})  [unwired: 1 in]
        n95 = Build Array(w229) -> (w236:cluster{sgl[], sgl[]}[])
      }
      frame "Idc" {
        n96 = Index Array(array=w248, index (col)=0 ("Index")) -> (element=w247:sgl[])  [unwired: 1 in]
        n97 = Index Array(array=w248, index (col)=2 ("Index")) -> (element=w244:sgl[])  [unwired: 1 in]
        n98 = Bundle("Data p1"=w245, "Data p1"=w254) -> ()  [unwired: 1 in, 1 out]
        n99 = Build Array (concatenate)(w244, w246) -> (w242:sgl[])
        n100 = Build Array (concatenate)(w247, w245) -> (w243:sgl[])
        n101 = Bundle(w243, w242) -> (w253:cluster{sgl[], sgl[]})  [unwired: 1 in]
        n102 = Build Array(w253) -> (w252:cluster{sgl[], sgl[]}[])
      }
      frame "E range" {
        n103 = Bundle("Data p1"=w263, "Data p1"=w259) -> (w262:cluster{"Data p1":sgl[], "Data p1":sgl[]})  [unwired: 1 in]
        n104 = Bundle("Data p1"=w263, "Data p1"=w260) -> ()  [unwired: 1 in, 1 out]
        n105 = Build Array(w262) -> (w261:cluster{"Data p1":sgl[], "Data p1":sgl[]}[])
      }
      frame "I range" {
        n106 = Bundle("Data p1"=w271, "Data p1"=w272) -> (w270:cluster{"Data p1":sgl[], "Data p1":sgl[]})  [unwired: 1 in]
        n107 = Build Array(w270) -> (w269:cluster{"Data p1":sgl[], "Data p1":sgl[]}[])
      }
      frame "f(t)" {
        n108 = Bundle("Data p1"=w281, "Data p1"=w280) -> (w279:cluster{"Data p1":sgl[], "Data p1":sgl[]})  [unwired: 1 in]
        n109 = Build Array(w279) -> (w278:cluster{"Data p1":sgl[], "Data p1":sgl[]}[])
      }
      frame "theta" {
        n110 = Divide(x=w290, y=6.283185307179586) -> (x/y=w292:dbl[])
        n111 = Divide(x=w298, y=6.283185307179586) -> (x/y=w301:dbl[])
        n112 = Multiply(x=w292, y=360) -> (x*y=w294:dbl[])
        n113 = Multiply(x=w301, y=360) -> (x*y=w297:dbl[])
        n114 = Bundle("Data p1"=w289, w297) -> (w288:cluster{"Data p1":sgl[], dbl[]})  [unwired: 1 in]
        n115 = Bundle("Data p1"=w289, w294) -> ()  [unwired: 1 in, 1 out]
        n116 = Build Array(w288) -> (w287:cluster{"Data p1":sgl[], dbl[]}[])
      }
    }
    "XY Graph" <- w122
    n117 = Array Size(array=w124) -> (size(s)=→"Number of points":i32)
    n118 = property on="XY Graph" class="XYGraph (strict)"("X Scale.Name Label.Text"=w157) -> ()  [unwired: 2 in, 2 out]
    n119 = property on="XY Graph" class="XYGraph (strict)"("Y Scale.Name Label.Text"=w160) -> ()  [unwired: 2 in, 2 out]
    n120 = property on="XY Graph" class="XYGraph (strict)"("Y Scale.Mapping Mode"=w145) -> ()  [unwired: 2 in, 2 out]
    n121 = local read "Exit 2"() -> (w153:bool)
    n122 = property on="XY Graph" class="XYGraph (strict)"("Y Scale.Flipped"=w155) -> ()  [unwired: 2 in, 2 out]
    n123 = property on="XY Graph" class="XYGraph (strict)"("X Scale.Mapping Mode"=w154) -> ()  [unwired: 2 in, 2 out]
  }
  n124 = call "disconnect.vi"("error in (no error)"=w11, "ID In"=w19) -> ("error out"=w8:errorcluster)  [unwired: 9 in]
  n125 = call <vilib>:"Simple Error Handler.vi"("error in (no error)"=w8) -> ()  [unwired: 4 in, 5 out]
